vi "Asylum_Driver_ExecuteLithographyObject.vi"(4 "Abort Notifier":refnum<notifier>, 6 "Interpolation":dbl format="%#_13g", 7 "Writing Setpoint":dbl=0.1 format="%#_13g", 8 "error in (no error)":errorcluster, 9 "Offsets":cluster{"X":dbl, "Y":dbl}, 10 "Pattern Data":T2={"Name"="", "Litho"=[], "Set Resistance"=enum."1G ohm", "Meta"=variant}, 11 "Application In":refnum<k7>) -> (0 "error out":errorcluster, 1 "Y":dbl[](array[numeric]), 2 "X":dbl[](array[numeric]), 3 "Application Out":refnum<k7>)   [LabVIEW 2019]
uses:
  <userlib>/LevyLab/Relay Box/Typedefs/Resistor--enum.ctl
  <userlib>/LevyLab/Relay Box/Relay-Box.lvclass
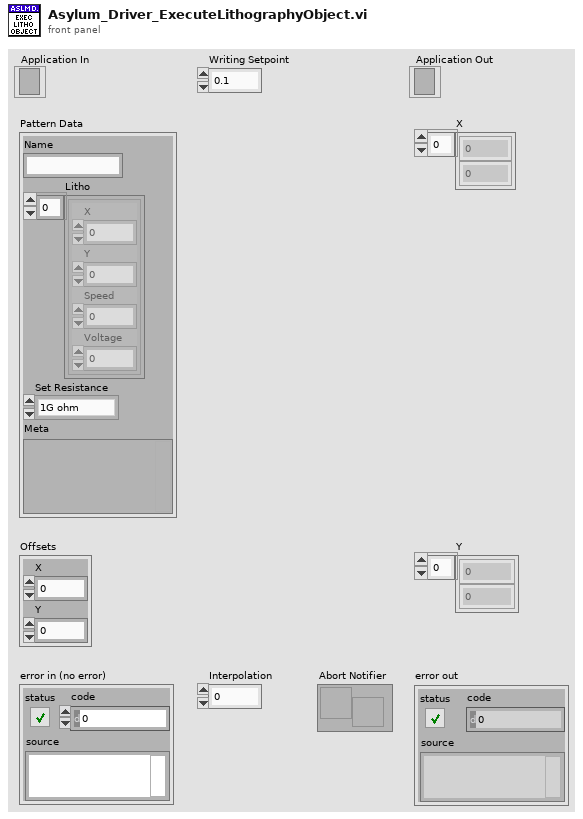
[diagram p1: front panel]
types:
  T1 = typedef "Relay-Box.lvclass/Resistor--enum.ctl" = enum16{"open", "discharge tip", "0 ohms", "100k ohm", "10M ohm", "1G ohm"}
  T2 = cluster{"Name":string, "Litho":cluster{"X":dbl, "Y":dbl, "Speed":dbl, "Voltage":dbl}[], "Set Resistance":T1, "Meta":variant}
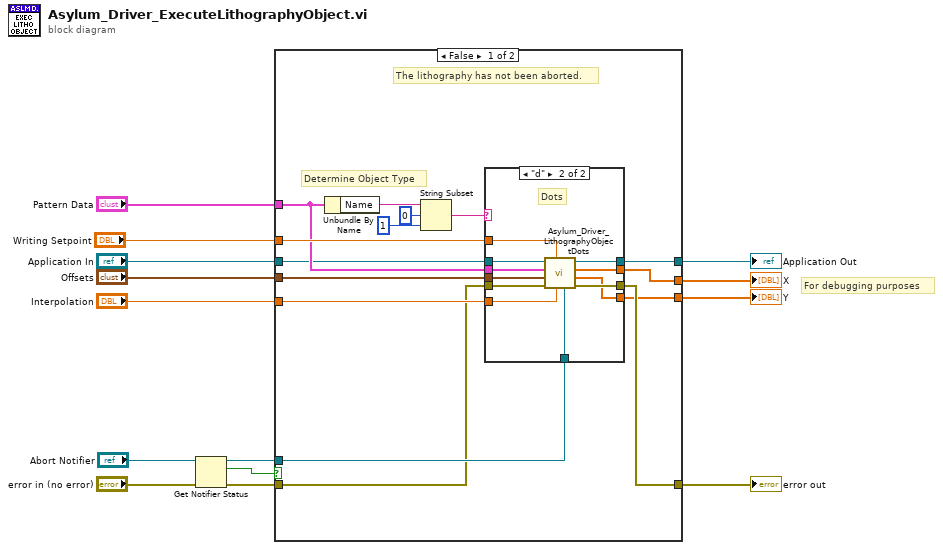
[diagram p0: block diagram]
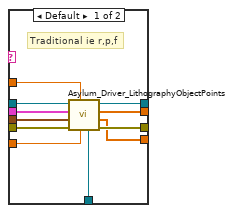
[diagram p2: hidden frame]
diagram:
  # "For debugging purposes"
  n1 = Get Notifier Status(notifier="Abort Notifier", error in (no error)="error in (no error)") -> (notifier out=w9:refnum<notifier>, current notification=w3:bool, error out=w12:errorcluster)  [unwired: 2 out]
  n2 = case shown="False" w3 {
    tunnel: w12 -> [w21 w52]
    tunnel: [w20 w52] -> w11
    tunnel: "Interpolation" -> [w29 _]
    tunnel: w9 -> [w28 _]
    tunnel: "Offsets" -> [w27 _]
    tunnel: "Pattern Data" -> [w25 _]
    tunnel: "Application In" -> [w19 w53]
    tunnel: [w18 w53] -> w5
    tunnel: "Writing Setpoint" -> [w26 _]
    tunnel: [w16 _] -> w2
    tunnel: [w15 _] -> w1
    frame False {
      # "The lithography has not been aborted."
      # "Determine Object Type"
      n3 = Unbundle By Name(w25) -> ("Name"=w24:string)
      n4 = String Subset(string=w24, offset (0)=0, length (rest)=1 ("length (rest)")) -> (substring=w17:string)
      n5 = case shown="\"d\"" w17 {
        tunnel: w29 -> [w40 w43]
        tunnel: w28 -> [w39 w47]
        tunnel: w27 -> [w38 w46]
        tunnel: w26 -> [w37 w44]
        tunnel: w25 -> [w36 w45]
        tunnel: w21 -> [w35 w48]
        tunnel: [w34 w49] -> w20
        tunnel: w19 -> [w33 w50]
        tunnel: [w32 w51] -> w18
        tunnel: [w31 w42] -> w16
        tunnel: [w30 w41] -> w15
        frame Default {
          # "Traditional ie r,p,f"
          n6 = call "Asylum_Driver_LithographyObjectPoints.vi"("Abort Notifier"=w39, "Interpolation"=w40, "Writing Setpoint"=w37, "error in (no error)"=w35, "Offsets"=w38, "Pattern Data"=w36, "Application"=w33) -> ("error out"=w34:errorcluster, "Y"=w30:dbl[], "X"=w31:dbl[], "Application"=w32:refnum<k7>)  [unwired: 1 in]
        }
        frame "d" {
          # "Dots"
          n7 = call "Asylum_Driver_LithographyObjectDots.vi"("Abort Notifier"=w47, "Interpolation"=w43, "Writing Setpoint"=w44, "error in (no error)"=w48, "Offsets"=w46, "Pattern Data"=w45, "Application"=w50) -> ("error out"=w49:errorcluster, "Y"=w41:dbl[], "X"=w42:dbl[], "Application"=w51:refnum<k7>)  [unwired: 1 in]
        }
      }
    }
    frame True {
      # "This has been aborted in early stage"
    }
  }
  "error out" <- w11
  "Application Out" <- w5
  "X" <- w2
  "Y" <- w1
